vi "ep_Initialize Ranges and Sensitivity (Multiple Lines).vi"(8 "error in (no error)":errorcluster, 10 "current channels":T1[](array[typedef]) {"physical channels"."channel phase" items=["Phase A (L1)", "Phase B (L2)", "Phase C (L3)", "Phase N (Neutral)"]}, 11 "voltage channels":T1[](array[typedef]) {"physical channels"."channel phase" items=["Phase A (L1)", "Phase B (L2)", "Phase C (L3)", "Phase N (Neutral)"]}) -> (0 "error out":errorcluster, 2 "voltage ranges":T3[](array[typedef]), 3 "voltage sensitivity":T4[](array[typedef]), 5 "current ranges":T3[](array[typedef]), 7 "current sensitivity":T4[](array[typedef]))   [LabVIEW 2014, in "NI_EP_Power Quality.lvlib"]
uses:
  <vilib>/addons/Electrical Power/PQ/NI_EP_Power Quality.lvlib
  <vilib>/addons/Electrical Power/PQ/Common/Controls/ep_Channel Sensitivity.ctl
  <vilib>/addons/Electrical Power/PQ/Common/Controls/ep_Channel Ranges.ctl
  <vilib>/addons/Electrical Power/PQ/Common/Controls/ep_Channels Config.ctl
  <vilib>/addons/Electrical Power/PQ/Common/Controls/ep_Channel Phase.ctl
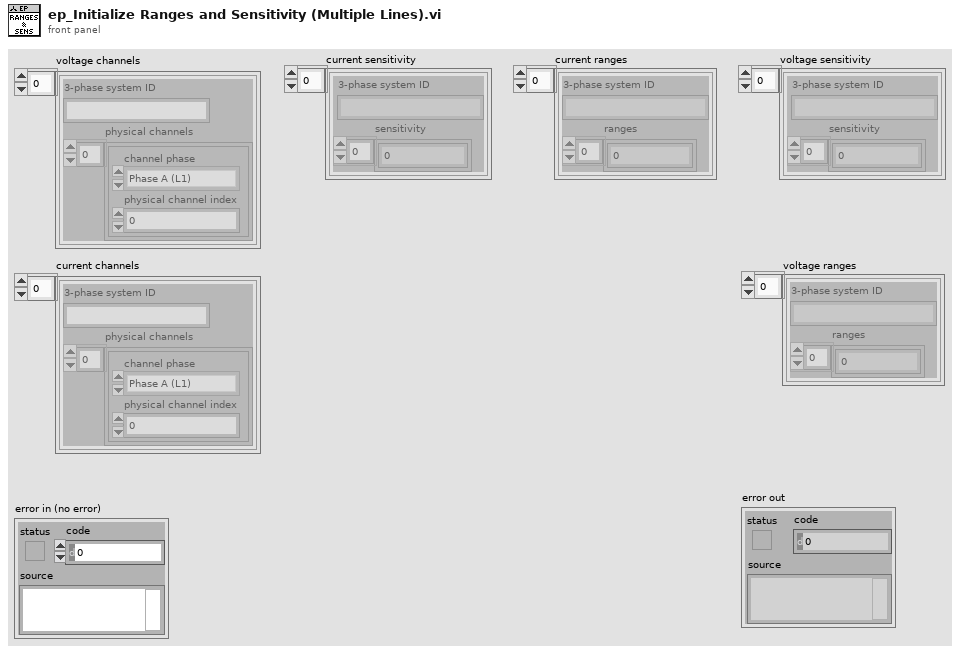
[diagram p1: front panel]
types:
  T1 = typedef "NI_EP_Power Quality.lvlib/ep_Channels Config.ctl" = cluster{"3-phase system ID":string, "physical channels":cluster{"channel phase":T2, "physical channel index":u16}[]}
  T2 = typedef "NI_EP_Power Quality.lvlib/ep_Channel Phase.ctl" = u16
  T3 = typedef "NI_EP_Power Quality.lvlib/ep_Channel Ranges.ctl" = cluster{"3-phase system ID":string, "ranges":dbl[]}
  T4 = typedef "NI_EP_Power Quality.lvlib/ep_Channel Sensitivity.ctl" = cluster{"3-phase system ID":string, "sensitivity":dbl[]}
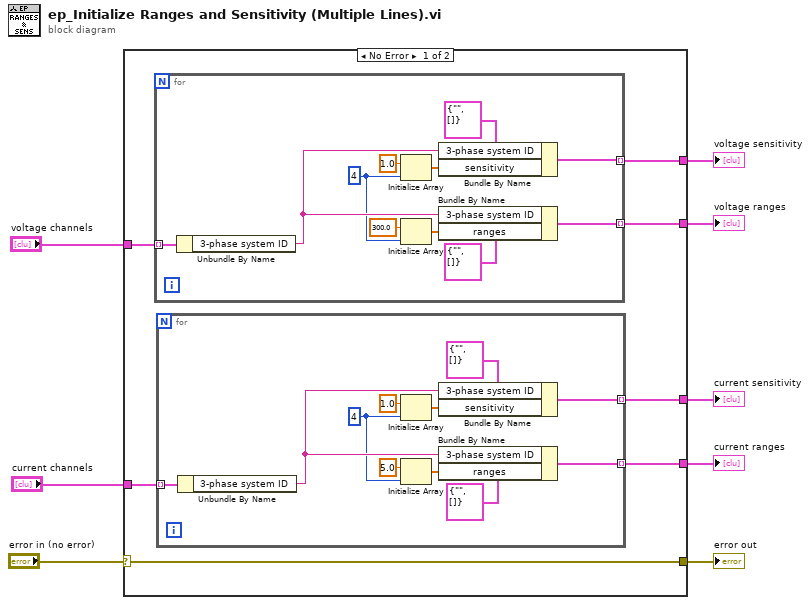
[diagram p0: block diagram]
diagram:
  n1 = case shown="No Error" "error in (no error)" {
    selector: "error in (no error)" -> [w13 w38]
    tunnel: "voltage channels" -> [w15 _]
    tunnel: "current channels" -> [w14 _]
    tunnel: [w10 _] -> w4
    tunnel: [w9 _] -> w3
    tunnel: [w13 w38] -> w7
    tunnel: [w12 _] -> w6
    tunnel: [w11 _] -> w5
    frame No Error {
      n2 = for {
        tunnel: w15 -> [w37] mode=indexing
        tunnel: [w28] -> w12 mode=indexing
        tunnel: [w27] -> w11 mode=indexing
        w29 = 4
        n3 = Unbundle By Name(w37) -> ("3-phase system ID"=w30:string)
        n4 = Initialize Array(1.0, w29) -> (w31:dbl[])
        n5 = Initialize Array(300.0, w29) -> (w34:dbl[])
        n6 = Bundle By Name(cluster=T4 {"3-phase system ID"="", "sensitivity"=[]} ("channel sensitivity"), "3-phase system ID"=w30, "sensitivity"=w31) -> (w28:T4)
        n7 = Bundle By Name(cluster=T3 {"3-phase system ID"="", "ranges"=[]} ("channel ranges"), "3-phase system ID"=w30, "ranges"=w34) -> (w27:T3)
      }
      n8 = for {
        tunnel: w14 -> [w26] mode=indexing
        tunnel: [w17] -> w10 mode=indexing
        tunnel: [w16] -> w9 mode=indexing
        w18 = 4
        n9 = Unbundle By Name(w26) -> ("3-phase system ID"=w19:string)
        n10 = Initialize Array(1.0, w18) -> (w20:dbl[])
        n11 = Initialize Array(5.0, w18) -> (w23:dbl[])
        n12 = Bundle By Name(cluster=T4 {"3-phase system ID"="", "sensitivity"=[]} ("channel sensitivity"), "3-phase system ID"=w19, "sensitivity"=w20) -> (w17:T4)
        n13 = Bundle By Name(cluster=T3 {"3-phase system ID"="", "ranges"=[]} ("channel ranges"), "3-phase system ID"=w19, "ranges"=w23) -> (w16:T3)
      }
    }
    frame Error {
    }
  }
  "voltage sensitivity" <- w6
  "voltage ranges" <- w5
  "current sensitivity" <- w4
  "current ranges" <- w3
  "error out" <- w7
